vi "Read Task File.vi"(8 "error in (no error)":errorcluster, 11 "IntanElectrophysiology in":refnum<class "IntanElectrophysiology.lvclass">) -> (0 "error out":errorcluster, 3 "IntanElectrophysiology out":refnum<class "IntanElectrophysiology.lvclass">)   [LabVIEW 2014, in "IntanElectrophysiology.lvclass"]
uses:
  IntanElectrophysiology.lvclass
  IntanElectrophysiology.lvclass/IntanElectrophysiology.ctl
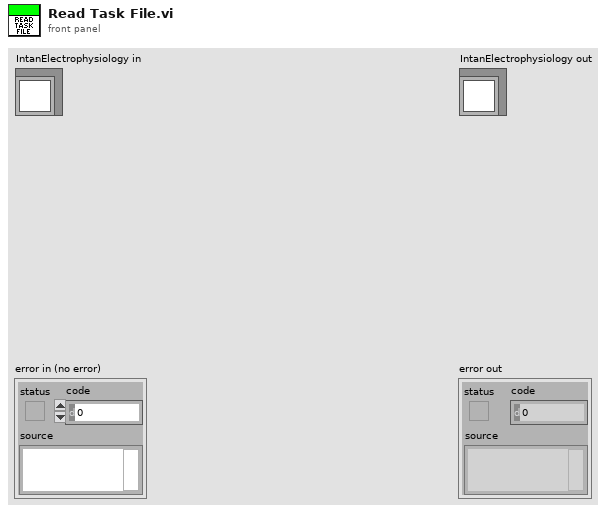
[diagram p1: front panel]
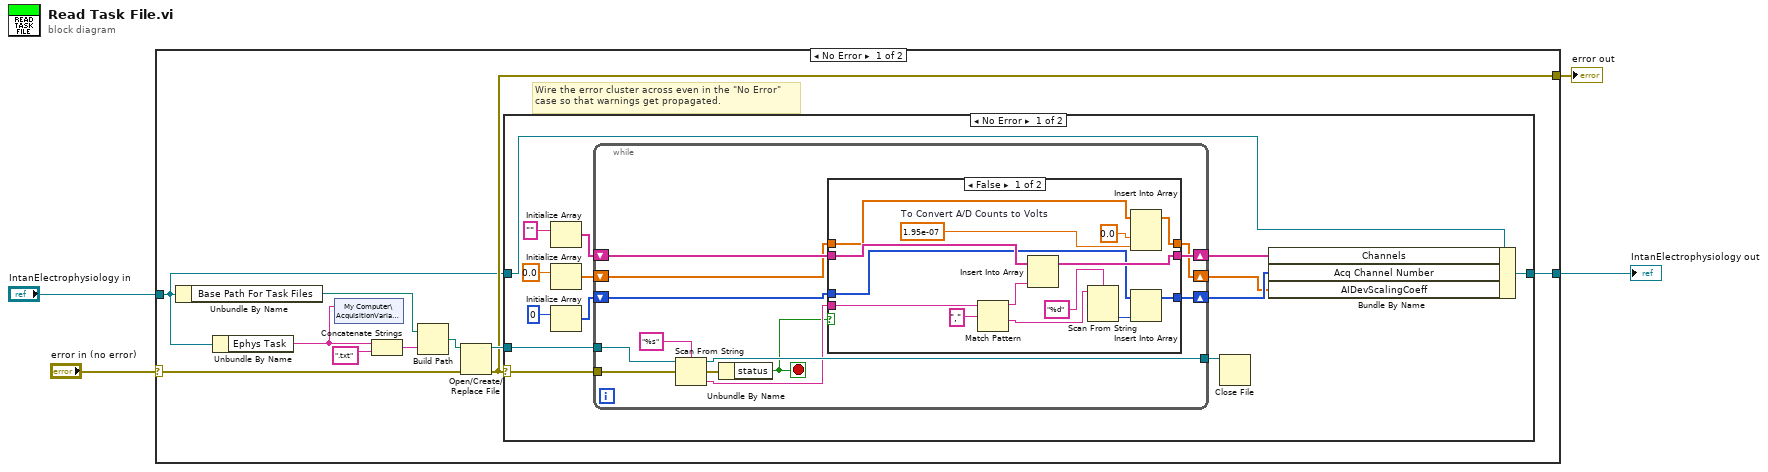
[diagram p0: block diagram]
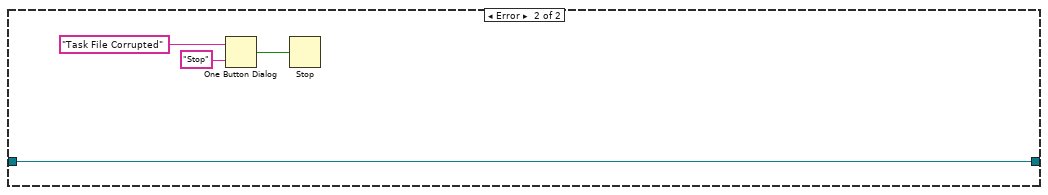
[diagram p3: hidden frame]
diagram:
  n1 = case shown="No Error" "error in (no error)" {
    selector: "error in (no error)" -> [w8 w64]
    tunnel: [w11 w64] -> w3
    tunnel: [w12 w63] -> w1
    tunnel: "IntanElectrophysiology in" -> [w9 w63]
    frame No Error {
      # "Wire the error cluster across even in the \"No Error\"\ncase so that warnings get propagated."
      n2 = Unbundle By Name(w9) -> ("Base Path For Task Files"=w10:path)
      n3 = Unbundle By Name(w9) -> ("Ephys Task"=w5:string)
      n4 = shared-variable "My Computer\\AcquisitionVariables.lvlib\\Task"(w5) -> ()  [unwired: 1 in, 1 out]
      n5 = Concatenate Strings(w5, ".txt" ("string")) -> (w6:string)
      n6 = Build Path(base path=w10, name or relative path=w6) -> (appended path=w14:path)
      n7 = Open/Create/Replace File(file path (use dialog)=w14, error in=w8) -> (refnum out=w13:refnum<file>, error out=w11:errorcluster)  [unwired: 4 in, 1 out]
      n8 = case shown="No Error" w11 {
        selector: w11 -> [w26 _]
        tunnel: w13 -> [w28 _]
        tunnel: w9 -> [w25 w59]
        tunnel: [w18 w59] -> w12
        frame No Error {
          n9 = Initialize Array("") -> (w22:string[])  [unwired: 1 in]
          n10 = Initialize Array(0.0 ("element")) -> (w16:dbl[])  [unwired: 1 in]
          n11 = Initialize Array(0 ("element")) -> (w21:i32[])  [unwired: 1 in]
          n12 = while {
            tunnel: w28 -> [w41]
            tunnel: [w39] -> w27
            tunnel: w26 -> [w38]
            shift-right: [w36] -> w20
            shift-left: w22 -> [w37]
            shift-right: [w34] -> w19
            shift-left: w21 -> [w35]
            shift-right: [w29] -> w15
            shift-left: w16 -> [w30]
            stop <- w31 stop-if-true
            n13 = Scan From String("%s" ("format string"), w41, w38) -> (w39:refnum<file>, w32:errorcluster, output 1=w33:string)  [unwired: 1 in]
            n14 = Unbundle By Name(w32) -> ("status"=w31:bool)
            n15 = case shown="False" w31 {
              tunnel: w37 -> [w55 w57]
              tunnel: [w54 w57] -> w36
              tunnel: w35 -> [w53 w58]
              tunnel: [w52 w58] -> w34
              tunnel: w33 -> [w51 _]
              tunnel: w30 -> [w45 w56]
              tunnel: [w44 w56] -> w29
              frame False {
                w43 = 1.95e-07  # To Convert A/D Counts to Volts
                n16 = Match Pattern(string=w51, regular expression=",") -> (before substring=w49:string, after substring=w48:string)  [unwired: 1 in, 2 out]
                n17 = Insert Into Array(array=w55, new element=w49) -> (w54:string[])  [unwired: 1 in]
                n18 = Scan From String(format string="%d", input string=w48) -> (output 1=w46:i32)  [unwired: 3 in, 3 out]
                n19 = Insert Into Array(array=w45, new element #1=0.0 ("new element/subarray"), new element #2=w43) -> (w44:dbl[])  [unwired: 1 in]
                n20 = Insert Into Array(array=w53, new element=w46) -> (w52:i32[])  [unwired: 1 in]
              }
              frame True {
              }
            }
          }
          n21 = Close File(refnum=w27) -> ()  [unwired: 1 in, 2 out]
          n22 = Bundle By Name(cluster=w25, "Channels"=w20, "Acq Channel Number"=w19, "AIDevScalingCoeff"=w15) -> (w18:refnum<class "IntanElectrophysiology.lvclass">)
        }
        frame Error {
          n23 = One Button Dialog(message="Task File Corrupted", button name ("OK")="Stop") -> (true=w60:bool)
          n24 = Stop(stop? (T)=w60) -> ()
        }
      }
    }
    frame Error {
    }
  }
  "error out" <- w3
  "IntanElectrophysiology out" <- w1
